vi "RotateTranslatePoints.vi"(10 "WaferAlignment":T1, 11 ".NET Refnum in":refnum<k24>) -> (2 "GetListData":refnum<k24>[](array[refnum]), 3 "Array":T2(array[cluster]))   [LabVIEW 2020]
uses:
  C:/Users/User/Desktop/Automation/CurrentVersion/LabviewDXFViewer/bin/Release/LabviewDXFViewer.exe
  LabviewDXFViewer/bin/Release/LabviewDXFViewer.exe
  WaferAlignmentType.ctl
  System.Drawing
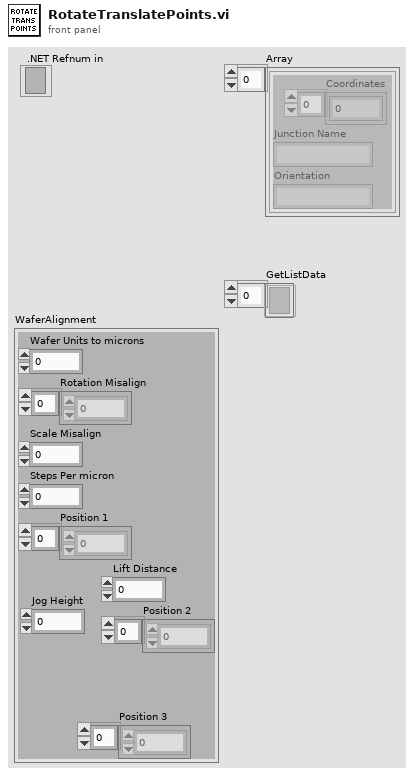
[diagram p1: front panel]
types:
  T1 = typedef "WaferAlignmentType.ctl" = cluster{"Wafer Units to microns":dbl, "Rotation Misalign":dbl[], "Scale Misalign":dbl, "Steps Per micron":dbl, "Position 1":i32[], "Position 2":i32[], "Lift Distance":i32, "Position 3":i32[], "Jog Height":i32}
  T2 = cluster{"Coordinates":dbl[], "Junction Name":string, "Orientation":string}[]
  T3 = cluster{"Coordinates":dbl[], "Junction Name":string, "Orientation":string}
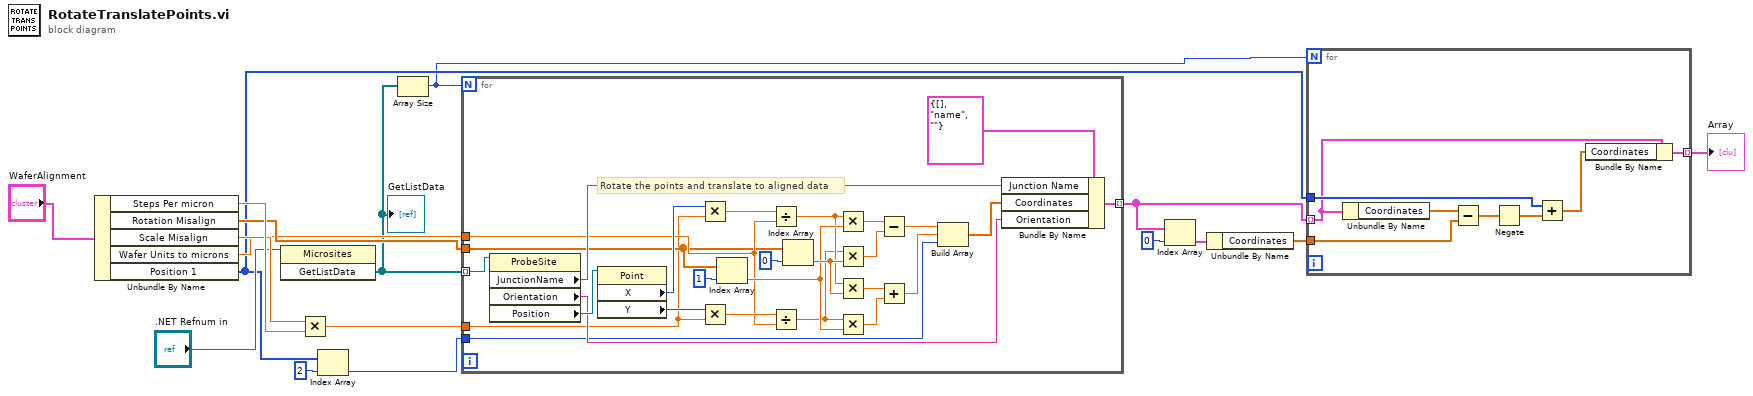
[diagram p0: block diagram]
diagram:
  n1 = Unbundle By Name("WaferAlignment") -> ("Steps Per micron"=w17:dbl, "Rotation Misalign"=w15:dbl[], "Scale Misalign"=w16:dbl, "Wafer Units to microns"=w14:dbl, "Position 1"=w3:i32[])
  n2 = invoke class="Microsites" method="GetListData"(reference=".NET Refnum in") -> ("GetListData"=w13:refnum<k24>[])  [unwired: 2 in, 2 out]
  "GetListData" <- w13
  n3 = Multiply(x=w16, y=w17) -> (x*y=w9:dbl)
  n4 = Index Array(array=w3, index=2) -> (element=w11:i32)
  n5 = Array Size(array=w13) -> (size(s)=w2:i32)
  n6 = for {
    N: w2 -> [_]
    tunnel: w13 -> [w43] mode=indexing
    tunnel: [w26] -> w5 mode=indexing
    tunnel: w14 -> [w21]
    tunnel: w15 -> [w20]
    tunnel: w9 -> [w19]
    tunnel: w11 -> [w18]
    # "Rotate the points and translate to aligned data"
    n7 = property class="ProbeSite"(reference=w43) -> ("JunctionName"=w28:string, "Orientation"=w27:string, "Position"=w44:refnum<k24>)  [unwired: 1 in, 2 out]
    n8 = property class="Point"(reference=w44) -> ("X"=w42:i32, "Y"=w41:i32)  [unwired: 1 in, 2 out]
    n9 = Multiply(x=w42, y=w19) -> (x*y=w24:dbl)
    n10 = Multiply(x=w41, y=w19) -> (x*y=w22:dbl)
    n11 = Index Array(array=w20, index=1) -> (element=w35:dbl)
    n12 = Divide(x=w24, y=w21) -> (x/y=w25:dbl)
    n13 = Divide(x=w22, y=w21) -> (x/y=w23:dbl)
    n14 = Index Array(array=w20, index=0) -> (element=w36:dbl)
    n15 = Multiply(x=w25, y=w35) -> (x*y=w38:dbl)
    n16 = Multiply(x=w23, y=w36) -> (x*y=w37:dbl)
    n17 = Multiply(x=w25, y=w36) -> (x*y=w34:dbl)
    n18 = Multiply(x=w23, y=w35) -> (x*y=w33:dbl)
    n19 = Subtract(x=w38, y=w37) -> (x-y=w32:dbl)
    n20 = Add(x=w34, y=w33) -> (x+y=w31:dbl)
    n21 = Build Array(w32, w31, w18) -> (w30:dbl[])
    n22 = Bundle By Name(cluster=T3 {"Coordinates"=[], "Junction Name"="name", "Orientation"=""} ("input cluster"), "Junction Name"=w28, "Coordinates"=w30, "Orientation"=w27) -> (w26:T3)
  }
  n23 = Index Array(array=w5, index=0) -> (element=w7:T3)
  n24 = Unbundle By Name(w7) -> ("Coordinates"=w6:dbl[])
  n25 = for {
    N: w2 -> [_]
    tunnel: w3 -> [w50]
    tunnel: w6 -> [w51]
    tunnel: w5 -> [w49] mode=indexing
    tunnel: [w47] -> w4 mode=indexing
    n26 = Unbundle By Name(w49) -> ("Coordinates"=w52:dbl[])
    n27 = Subtract(x=w52, y=w51) -> (x-y=w46:dbl[])
    n28 = Negate(x=w46) -> (-x=w45:dbl[])
    n29 = Add(x=w50, y=w45) -> (x+y=w48:dbl[])
    n30 = Bundle By Name(cluster=w49, "Coordinates"=w48) -> (w47:T3)
  }
  "Array" <- w4
